vi "Kinect Test1.vi"() -> ()   [LabVIEW 2014]
uses:
  <vilib>/University of Leeds/Kinesthesia Toolkit for Microsoft Kinect/_Polymorphic Configure/Event-Depth, Skeleton and Video.vi
  <vilib>/University of Leeds/Kinesthesia Toolkit for Microsoft Kinect/_Polymorphic Read/Read-Depth, Skeleton and Video.vi
  <vilib>/University of Leeds/Kinesthesia Toolkit for Microsoft Kinect/_Polymorphic Close/Close-Depth, Skeleton and Video.vi
panel:
  out "3D Picture":refnum<vi>(3d-picture)
  out "new picture 2":picture
  out "new picture":picture
  out "Render 3S Skeleton error":errorcluster
  out "Read error":errorcluster
  in  "stop":bool
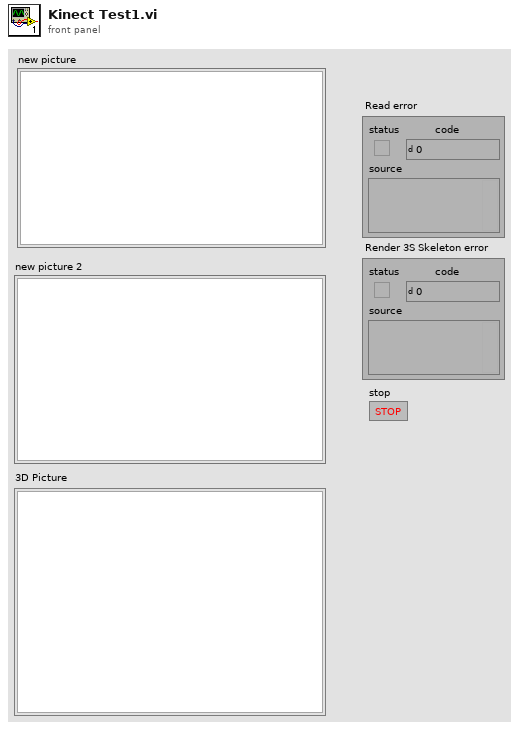
[diagram p1: front panel]
types:
  T1 = cluster{cluster{"reference out":refnum<k24>, "KinectSensors":refnum<k24>}, "get_Item":refnum<k24>}
  T2 = cluster{"reference out":refnum<k24>, "KinectSensors":refnum<k24>, "SkeletonStream":refnum<k24>, "DepthStream":refnum<k24>, "ColorStream":refnum<k24>, refnum<k24>[], "get_Item":refnum<k24>}
  T3 = cluster{"Scene":refnum<vi>, "Joints":refnum<vi>[], "Bones":refnum<vi>[]}
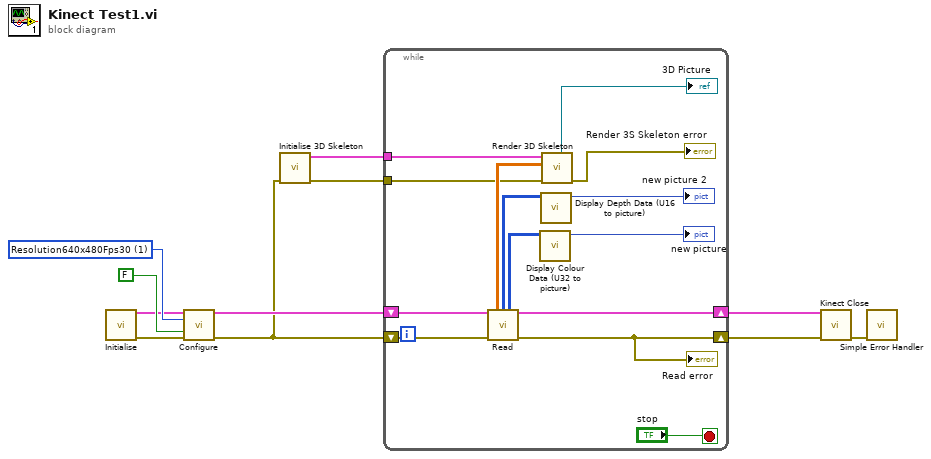
[diagram p0: block diagram]
diagram:
  w9 = 1 items=["Undefined", "Resolution640x480Fps30", "Resolution320x240Fps30", "Resolution80x60Fps30"] ("Depth Stream Format")
  n1 = call <vilib>:"Initialise.vi"() -> ("Kinect References out"=w7:T1, "error out"=w11:errorcluster)  [unwired: 14 in]
  n2 = call-poly <vilib>:"Configure.vi"("Kinect References in"=w7, "Depth Stream Format"=w9, "Skeleton Smoothing"=FALSE, "error in"=w11) -> ("Kinect References out"=w6:T2, "error out"=w2:errorcluster)  [unwired: 10 in]
  n3 = call <vilib>:"Initialise 3D Skeleton.vi"("error in (no error)"=w2) -> ("error out"=w3:errorcluster, "Scene & Skeleton Refs"=w4:T3)  [unwired: 9 in]
  n4 = while {
    shift-right: [w24] -> w10
    shift-left: w2 -> [w25]
    shift-right: [w23] -> w5
    shift-left: w6 -> [w22]
    tunnel: w4 -> [w18]
    tunnel: w3 -> [w17]
    stop <- "stop" stop-if-true
    n5 = call-poly <vilib>:"Read.vi"("Kinect References in"=w22, "error in (no error)"=w25) -> ("Primary Skeleton Array"=w19:dbl[][], "Depth output array (U16)"=w21:u16[][], "Colour output array (U24, RGB)"=w20:u32[][], "Kinect References out"=w23:T2, "error out"=w24:errorcluster)  [unwired: 8 in, 1 out]
    "Read error" <- w24
    n6 = call <vilib>:"Display Colour Data (U32 to picture).vi"("Colour output array (U24, RGB)"=w20) -> ("new picture"=→"new picture":picture)  [unwired: 10 in]
    n7 = call <vilib>:"Display Depth Data (U16 to picture).vi"("Depth output array (U16)"=w21) -> ("new picture"=→"new picture 2":picture)  [unwired: 10 in]
    n8 = call <vilib>:"Render 3D Skeleton.vi"("error in (no error)"=w17, "Array of Joint Positions"=w19, "Scene & Skeleton Refs In"=w18) -> ("error out"=→"Render 3S Skeleton error":errorcluster, "Scene Out"=→"3D Picture":refnum<vi>)  [unwired: 5 in, 2 out]
  }
  n9 = call-poly <vilib>:"Kinect Close.vi"("Kinect References in"=w5, "error in"=w10) -> ("error out"=w1:errorcluster)  [unwired: 13 in]
  n10 = call <vilib>:"Simple Error Handler.vi"("error in (no error)"=w1) -> ()  [unwired: 4 in, 5 out]
